vi "GetWireTerminalByType__slk_mt.vi"(8 "error in (no error)":errorcluster, 11 "wire refnum in":refnum<vi>) -> (0 "error out":errorcluster, 1 "sink terminals out":refnum<vi>[](array[refnum]), 2 "source terminal out":refnum<vi>, 3 "duplicated wire refnum out":refnum<vi>)   [LabVIEW 2020]
doc: "Returns the terminals with specified wire by type (source or sink)."
panel:
  # "GetWireTerminalByType__slk_mt.vi\nReturns the terminals with specified wire by type (source or sink).\n\nNOTICE -- YOU MUST LEAVE THIS NOTICE IN PLACE.\n\nCopyright (c) 2011, LIANG LIU Shawn.Liu.cn@gmail.com\nAll rights reserved.\n\nRedistribution and use in source and binary forms, with or without modification, are permitted provided that the following conditions are met:\n-Redistributions of source code must retain the above copyright notice, this list of conditions and the following disclaimer.\n-Redistributions in binary form must reproduce the above copyright notice, this list of conditions and the following disclaimer in the documentation and/or other materials provided with the distribution.\n-Neither the name of the eLp nor the names of its contributors may be used to endorse or promote products derived from this software without specific prior written permission.\n\nTHIS SOFTWARE IS PROVIDED BY THE COPYRIGHT HOLDERS AND CONTRIBUTORS \"AS IS\" AND ANY EXPRESS OR IMPLIED WARRANTIES, INCLUDING, BUT NOT LIMITED TO, THE IMPLIED WARRANTIES OF MERCHANTABILITY AND FITNESS FOR A PARTICULAR PURPOSE ARE DISCLAIMED. IN NO EVENT SHALL THE COPYRIGHT HOLDER OR CONTRIBUTORS BE LIABLE FOR ANY DIRECT, INDIRECT, INCIDENTAL, SPECIAL, EXEMPLARY, OR CONSEQUENTIAL DAMAGES (INCLUDING, BUT NOT LIMITED TO, PROCUREMENT OF SUBSTITUTE GOODS OR SERVICES; LOSS OF USE, DATA, OR PROFITS; OR BUSINESS INTERRUPTION) HOWEVER CAUSED AND ON ANY THEORY OF LIABILITY, WHETHER IN CONTRACT, STRICT LIABILITY, OR TORT (INCLUDING NEGLIGENCE OR OTHERWISE) ARISING IN ANY WAY OUT OF THE USE OF THIS SOFTWARE, EVEN IF ADVISED OF THE POSSIBILITY OF SUCH DAMAGE."
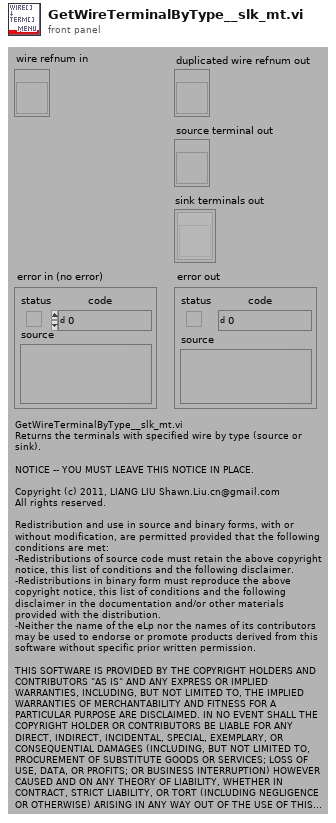
[diagram p1: front panel]
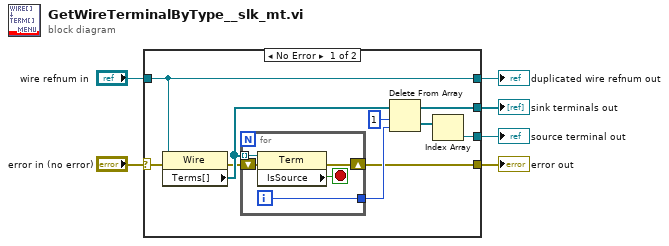
[diagram p0: block diagram]
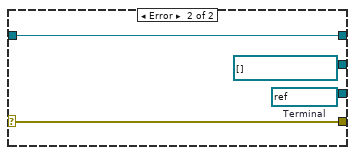
[diagram p2: hidden frame]
diagram:
  n1 = case shown="No Error" "error in (no error)" {
    selector: "error in (no error)" -> [w8 w23]
    tunnel: [w12 w24] -> w6
    tunnel: [w11 refnum<vi>[] [] ("Terms[]")] -> w5
    tunnel: [w9 w23] -> w4
    tunnel: "wire refnum in" -> [w7 w22]
    tunnel: [w7 w22] -> w1
    frame No Error {
      n2 = property class="Wire"(reference=w7, error in=w8) -> (error out=w10:errorcluster, "Terms[]"=w16:refnum<vi>[])  [unwired: 1 out]
      n3 = for {
        tunnel: w16 -> [w21] mode=indexing
        tunnel: [w19] -> w15
        shift-right: [w17] -> w9
        shift-left: w10 -> [w18]
        i -> [w19]
        stop <- w20 stop-if-true
        n4 = property class="Term"(reference=w21, error in=w18) -> (error out=w17:errorcluster, "IsSource"=w20:bool)  [unwired: 1 out]
      }
      n5 = Delete From Array(array=w16, length=1, index=w15) -> (deleted portion=w13:refnum<vi>[], array with subset deleted=w11:refnum<vi>[])
      n6 = Index Array(array=w13) -> (element=w12:refnum<vi>)  [unwired: 1 in]
    }
    frame Error {
      w24 = refnum<vi> refnum  # Terminal
    }
  }
  "source terminal out" <- w6
  "sink terminals out" <- w5
  "duplicated wire refnum out" <- w1
  "error out" <- w4
